vi "打开数据库.vi"(0 "Display State In":T1={"扫描参数"={"+ V"=0.0, "+ Δ V"=0.0, "+ limit I"=0.01, "- V"=0.0, "- Δ V"=0.0, "- limit I"=0.01, "ΔT"=0.0, "NPLC"=0.001}, "保持时间"={"+ V"=0.0, "+ limit I"=0.01, "T"=0.0, "ΔT"=0.0, "NPLC"=0.001}, "功能选择"=enum."扫描", "强制时序"=FALSE, "数据库引用"=refnum} caption="显示状态输入" {"保持时间"."ΔT" format="%#_6ps"; "保持时间"."T" format="%#_6ps"; "保持时间"."NPLC" min=0.001 max=25.0 step=0.001; "保持时间"."+ limit I" min=1e-08 max=3.0 format="%#_6pA"; "保持时间"."+ V" min=-40.0 max=40.0 format="%#_6pV"; "扫描参数"."NPLC" min=0.001 max=25.0 step=0.001; "扫描参数"."- Δ V" min=0.0 max=1.0 format="%#_6pV"; "扫描参数"."+ Δ V" min=0.0 max=1.0 format="%#_6pV"; "扫描参数"."- V" min=-40.0 max=40.0 format="%#_6pV"; "扫描参数"."- limit I" min=1e-08 max=3.0 format="%#_6pA"; "扫描参数"."ΔT" format="%#_6ps"; "扫描参数"."+ limit I" min=1e-08 max=3.0 format="%#_6pA"; "扫描参数"."+ V" min=-40.0 max=40.0 format="%#_6pV"}, 5 "文件路径":path=path "D:/Data/Database.accdb", 9 "Container State":T6 caption="容器状态", 11 "error in (no error)":errorcluster caption="错误输入（无错误）") -> (4 "Display State Out":T1={"扫描参数"={"+ V"=0.0, "+ Δ V"=0.0, "+ limit I"=0.01, "- V"=0.0, "- Δ V"=0.0, "- limit I"=0.01, "ΔT"=0.0, "NPLC"=0.001}, "保持时间"={"+ V"=0.0, "+ limit I"=0.01, "T"=0.0, "ΔT"=0.0, "NPLC"=0.001}, "功能选择"=enum."扫描", "强制时序"=FALSE, "数据库引用"=refnum} caption="显示状态输出" {"保持时间"."ΔT" format="%#_6ps"; "保持时间"."T" format="%#_6ps"; "保持时间"."NPLC" min=0.001 max=25.0 step=0.001; "保持时间"."+ limit I" min=1e-08 max=3.0 format="%#_6pA"; "保持时间"."+ V" min=-40.0 max=40.0 format="%#_6pV"; "扫描参数"."NPLC" min=0.001 max=25.0 step=0.001; "扫描参数"."- Δ V" min=0.0 max=1.0 format="%#_6pV"; "扫描参数"."+ Δ V" min=0.0 max=1.0 format="%#_6pV"; "扫描参数"."- V" min=-40.0 max=40.0 format="%#_6pV"; "扫描参数"."- limit I" min=1e-08 max=3.0 format="%#_6pA"; "扫描参数"."ΔT" format="%#_6ps"; "扫描参数"."+ limit I" min=1e-08 max=3.0 format="%#_6pA"; "扫描参数"."+ V" min=-40.0 max=40.0 format="%#_6pV"}, 15 "error out":errorcluster caption="错误输出")   [LabVIEW 2020, in "功能选择.xctl"]
uses:
  <vilib>/_xctls/Container State.ctl
  <vilib>/addons/database/Connection.llb/Conn ObjectReference.ctl
  <vilib>/addons/database/Connection.llb/DB Tools Open Connec (String).vi
  <vilib>/addons/database/NI_Database_API.lvlib
  <vilib>/_xctls/XControlSupport.lvlib
panel:
  # "添加构成方法参数的输入控件及显示控件。连接至连线板。不要删除已连接至连线板的输入控件及显示控件。\n\n如需设置该方法的参数，右键单击项目树中的对应项并选择“配置方法...”。"
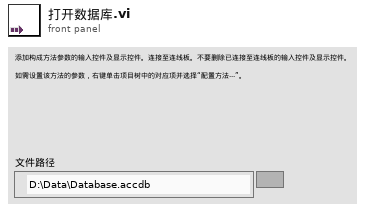
[diagram p1: front panel]
types:
  T1 = typedef "功能选择.xctl/状态.ctl" = cluster{"扫描参数":T2, "保持时间":T3, "功能选择":T4, "强制时序":bool, "数据库引用":T5}
  T2 = typedef "功能选择.xctl/扫描参数.ctl" = cluster{"+ V":dbl, "+ Δ V":dbl, "+ limit I":dbl, "- V":dbl, "- Δ V":dbl, "- limit I":dbl, "ΔT":dbl, "NPLC":dbl}
  T3 = typedef "功能选择.xctl/保持时间.ctl" = cluster{"+ V":dbl, "+ limit I":dbl, "T":dbl, "ΔT":dbl, "NPLC":dbl}
  T4 = typedef "功能选择.xctl/数据.ctl" = enum16{"扫描", "保持时间", "脉冲", "高速脉冲", "任意波形"}
  T5 = typedef "NI_Database_API.lvlib/Conn ObjectReference.ctl" = refnum<k1>
  T6 = typedef "XControlSupport.lvlib/Container State.ctl" = cluster{"Indicator?":bool, "Run Mode?":bool, " Refnum":refnum<vi>}
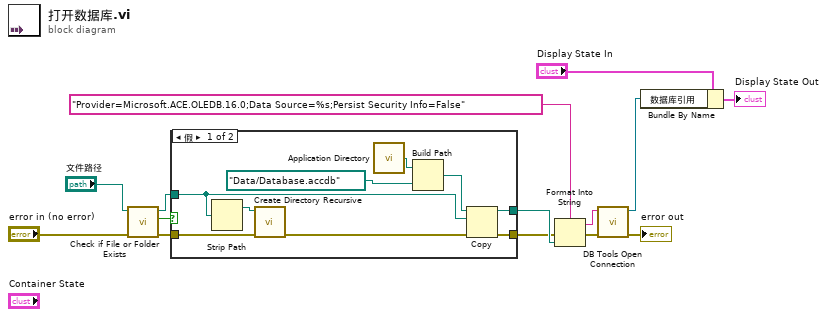
[diagram p0: block diagram]
diagram:
  n1 = call <vilib>:"Check if File or Folder Exists.vi"("error in (no error)"="error in (no error)", "path"="文件路径") -> ("error out"=w7:errorcluster, "file or folder exists?"=w12:bool, "dup path"=w11:path)  [unwired: 7 in]
  n2 = case shown="假" w12 {
    tunnel: w11 -> [w19 w25]
    tunnel: [w23 w25] -> w9
    tunnel: w7 -> [w20 w24]
    tunnel: [w22 w24] -> w6
    frame False {
      n3 = Strip Path(path=w19) -> (stripped path=w18:path)  [unwired: 1 out]
      n4 = call <vilib>:"Create Directory Recursive.vi"("error in (no error)"=w20, "directory"=w18) -> ("error out"=w21:errorcluster)  [unwired: 3 in, 2 out]
      n5 = call <vilib>:"Application Directory.vi"() -> ("Application Directory"=w17:path)
      n6 = Build Path(base path=w17, name or relative path=path "Data/Database.accdb" ("文件路径")) -> (appended path=w15:path)
      n7 = Copy(8:w21, 10:w19, 11:w15) -> (0:w22:errorcluster, 3:w23:path)  [unwired: 2 in, 1 out]
    }
    frame True {
    }
  }
  n8 = Format Into String(format string="Provider=Microsoft.ACE.OLEDB.16.0;Data Source=%s;Persist Security Info=False", error in=w6, w9) -> (resulting string=w8:string, error out=w5:errorcluster)  [unwired: 1 in]
  n9 = call-poly <vilib>:"DB Tools Open Connection.vi"("error in (no error)"=w5, "connection information"=w8) -> ("error out"=→"error out":errorcluster, "connection reference"=w1:T5)  [unwired: 6 in]
  n10 = Bundle By Name(cluster="Display State In", "数据库引用"=w1) -> (→"Display State Out":T1)
